vi "Value Multiple Numeric Controls.vi"(8 "error in (no error)":errorcluster, 10 "Value":dbl, 11 "References":refnum<vi>[](array[refnum])) -> (0 "error out":errorcluster)   [LabVIEW 2015]
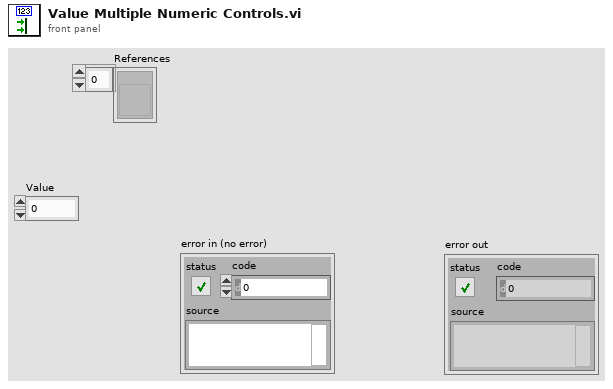
[diagram p1: front panel]
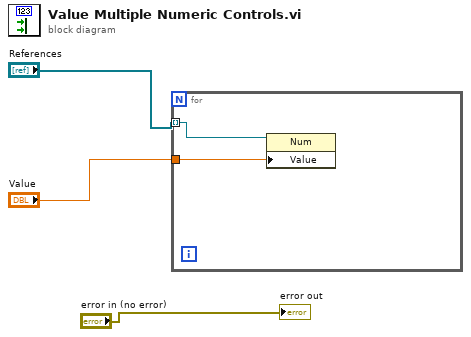
[diagram p0: block diagram]
diagram:
  n1 = for {
    tunnel: "References" -> [w5] mode=indexing
    tunnel: "Value" -> [w4]
    n2 = property class="Num"(reference=w5, "Value"=w4) -> ()  [unwired: 1 in, 2 out]
  }
  "error out" <- "error in (no error)"
